vi "Read port.vi"(8 "error in (no error)":errorcluster, 11 "MelsecTCP in":refnum<class "InovanceTCP.lvclass">) -> (0 "error out":errorcluster, 2 "port":i32, 3 "MelsecTCP out":refnum<class "InovanceTCP.lvclass">)   [LabVIEW 2020, in "HslCommunication.lvlib" / "InovanceTCP.lvclass"]
uses:
  InovanceTCP.lvclass
  InovanceTCP.lvclass/InovanceTCP.ctl
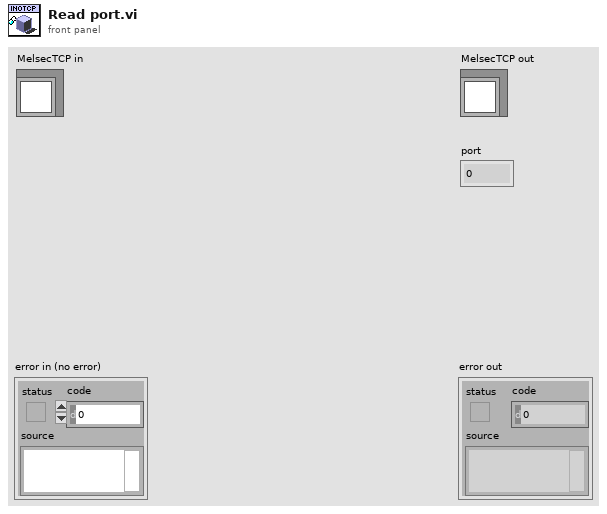
[diagram p1: front panel]
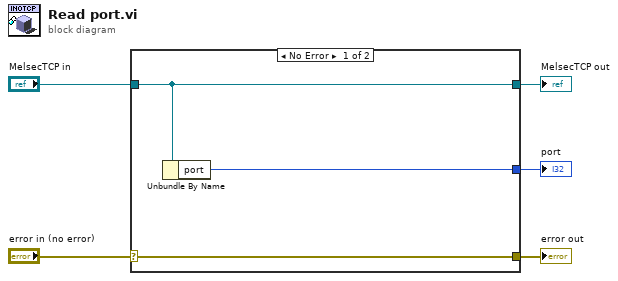
[diagram p0: block diagram]
diagram:
  n1 = case shown="No Error" "error in (no error)" {
    selector: "error in (no error)" -> [w8 w9]
    tunnel: [w8 w9] -> w4
    tunnel: [w7 w10] -> w2
    tunnel: "MelsecTCP in" -> [w7 w10]
    tunnel: [w6 _] -> w1
    frame No Error {
      n2 = Unbundle By Name(w7) -> ("port"=w6:i32)
    }
    frame Error {
    }
  }
  "error out" <- w4
  "MelsecTCP out" <- w2
  "port" <- w1
